vi "ElectrodeTest.vi"() -> ()   [LabVIEW 2014]
uses:
  Electrode XCtl/Electrode XCtl Folder/Electrode XCtl.xctl
panel:
  in  "Numeric":i32
  out "Electrode XCtl 2":T1(xcontrol)
  in  "String":string
  in  "Boolean":bool
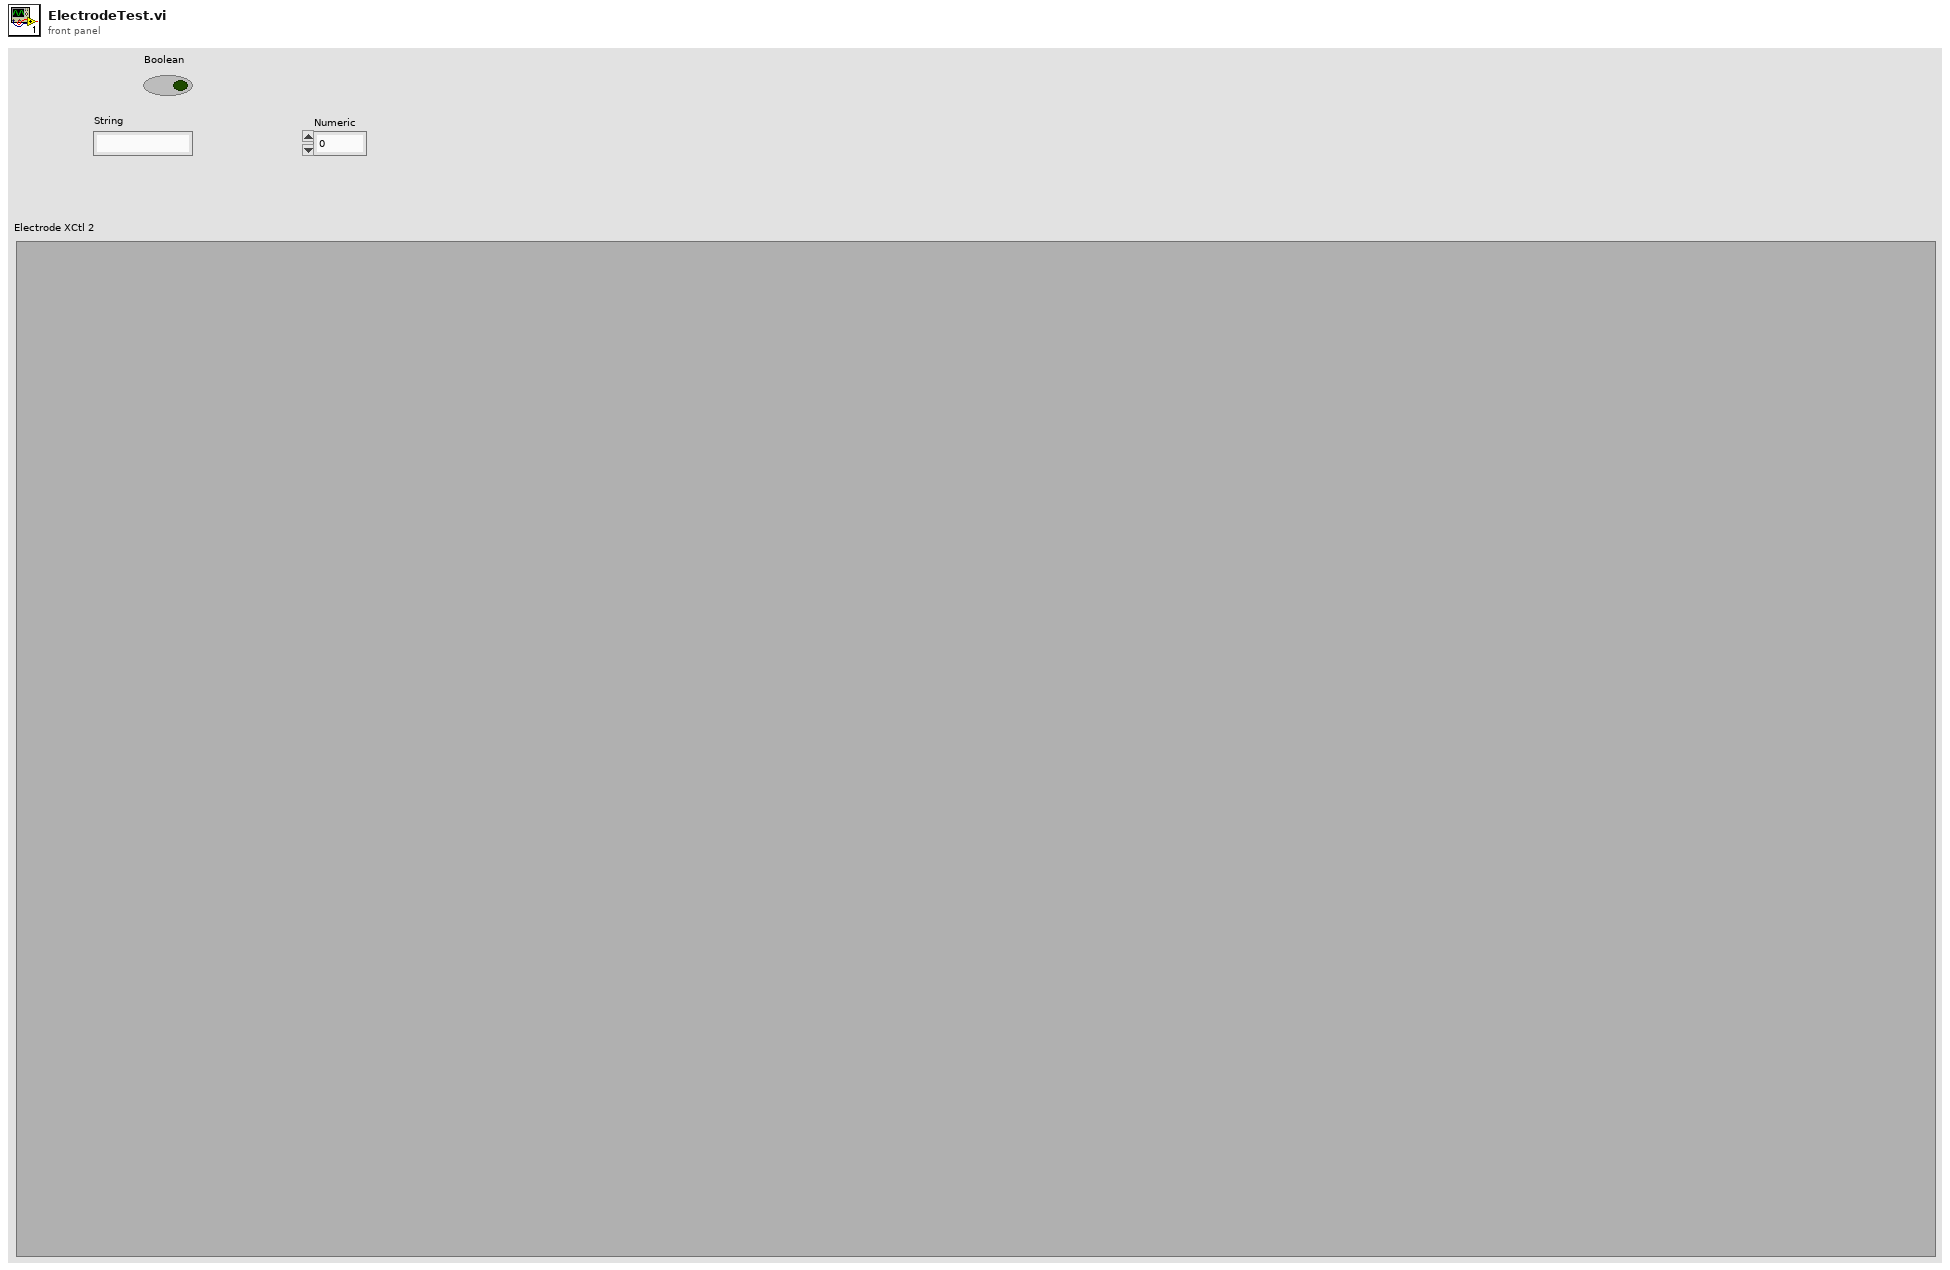
[diagram p1: front panel]
types:
  T1 = cluster{"Data":u16, "ElectrodeStates":cluster{"On_Off":bool, "Text":string}[], "ModOn":bool}
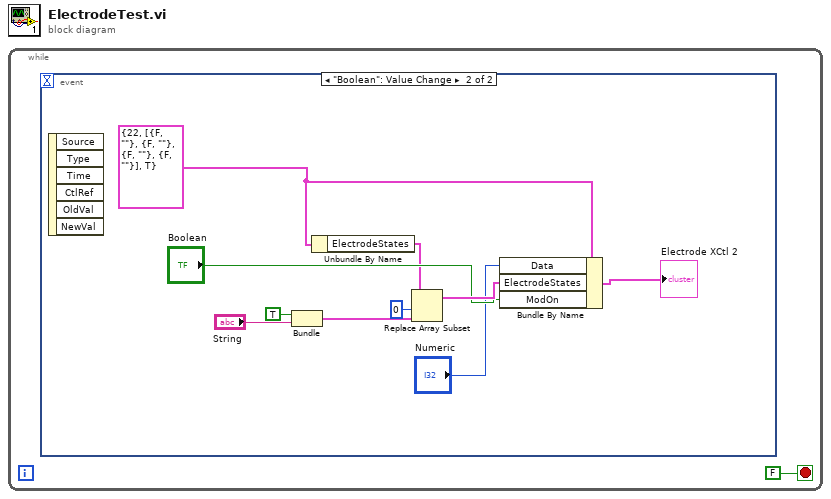
[diagram p0: block diagram]
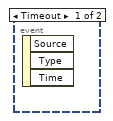
[diagram p2: hidden frame]
diagram:
  n1 = while {
    stop <- FALSE stop-if-true
    n2 = event shown="[1] \"Boolean\": Value Change" {
      selector: _ -> [_ _]
      dyn-events: _ -> [_ _]
      timeout: _ -> [_ _]
      event Timeout {
        n3 = event-data() -> ()  [unwired: 1 in, 3 out]
      }
      event "Boolean": Value Change {
        w2 = T1 {"Data"=22, "ElectrodeStates"=[{"On_Off"=FALSE, "Text"=""}, {"On_Off"=FALSE, "Text"=""}, {"On_Off"=FALSE, "Text"=""}, {"On_Off"=FALSE, "Text"=""}], "ModOn"=TRUE} ("Electrode XCtl")
        n4 = event-data() -> ()  [unwired: 1 in, 6 out]
        n5 = Bundle(TRUE, "String"="String") -> (w10:cluster{bool, "String":string})  [unwired: 1 in]
        n6 = Unbundle By Name(w2) -> ("ElectrodeStates"=w3:cluster{"On_Off":bool, "Text":string}[])
        n7 = Replace Array Subset(array=w3, new element=w10, index=0) -> (w9:cluster{"On_Off":bool, "Text":string}[])
        n8 = Bundle By Name(cluster=w2, "Data"="Numeric", "ElectrodeStates"=w9, "ModOn"="Boolean") -> (→"Electrode XCtl 2":T1)
      }
    }
  }
